vi "HackRF_Open.vi"(8 "error in (no error)":errorcluster, 11 "Device number":i32) -> (0 "error out":errorcluster, 3 "Cluster":T1)   [LabVIEW 2021]
uses:
  Users/fl1ckje/Downloads/LV_HackRF_FMreceiver-main/HackRF_Lib/HackRF_Ref.ctl
  C:/Users/fl1ckje/Downloads/LV_HackRF_FMreceiver-main/HackRF_Lib/NetHackrf.dll
  Users/fl1ckje/Downloads/LV_HackRF_FMreceiver-main/HackRF_Lib/NetHackrf.dll
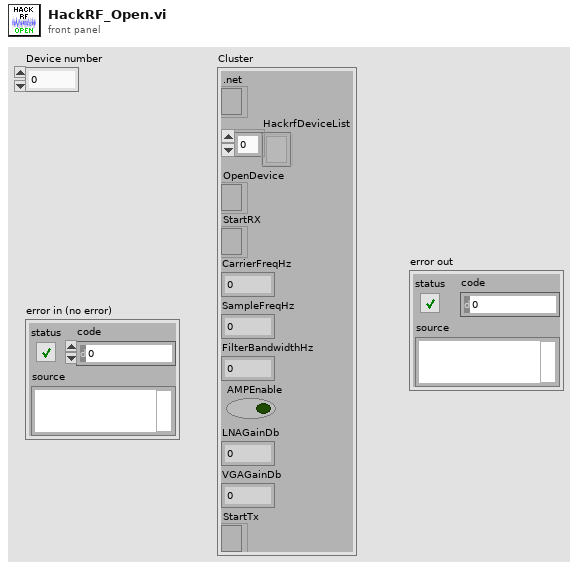
[diagram p1: front panel]
types:
  T1 = typedef "HackRF_Ref.ctl" = cluster{".net":refnum<k24>, "HackrfDeviceList":refnum<k24>[], "OpenDevice":refnum<k24>, "StartRX":refnum<k24>, "CarrierFreqHz":dbl, "SampleFreqHz":dbl, "FilterBandwidthHz":dbl, "AMPEnable":bool, "LNAGainDb":dbl, "VGAGainDb":dbl, "StartTx":refnum<k24>}
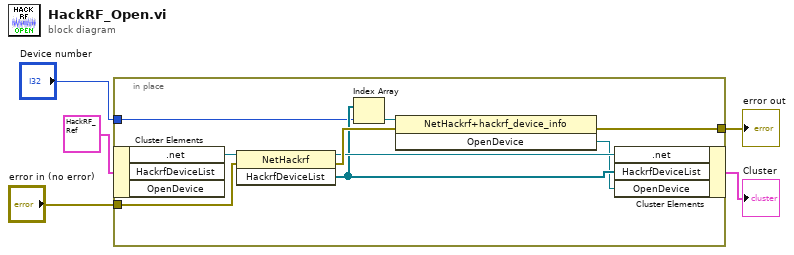
[diagram p0: block diagram]
diagram:
  n1 = in-place {
    in-place-border: "Device number" -> [w8]
    in-place-border: "error in (no error)" -> [w7]
    in-place-border: [w6] -> w4
    n2 = in-place-cluster #1(T1 {".net"=refnum, "HackrfDeviceList"=[], "OpenDevice"=refnum, "StartRX"=refnum, "CarrierFreqHz"=0.0, "SampleFreqHz"=0.0, "FilterBandwidthHz"=0.0, "AMPEnable"=FALSE, "LNAGainDb"=0.0, "VGAGainDb"=0.0, "StartTx"=refnum}) -> (".net"=w12:refnum<k24>)  [unwired: 2 out]
    n3 = invoke class="NetHackrf" method="HackrfDeviceList"(reference=w12, error in=w7) -> (reference out=w11:refnum<k24>, error out=w13:errorcluster, "HackrfDeviceList"=w10:refnum<k24>[])  [unwired: 1 in]
    n4 = Index Array(array=w10, index=w8) -> (element=w14:refnum<k24>)
    n5 = invoke class="NetHackrf+hackrf_device_info" method="OpenDevice"(reference=w14, error in=w13) -> (error out=w6:errorcluster, "OpenDevice"=w9:refnum<k24>)  [unwired: 1 in, 1 out]
    n6 = in-place-cluster #1(".net"=w11, "HackrfDeviceList"=w10, "OpenDevice"=w9) -> (→"Cluster":T1)
  }
  "error out" <- w4
